vi "NavX Init.vi"(8 "error in":errorcluster) -> (0 "error out":errorcluster)   [LabVIEW 2015]
uses:
  <vilib>/Rock Robotics/SystemInterfaces/spilib/spi_bus.ctl
  Support/Global Objects.vi
  navX Library v2/IO/Open/Z900_navX_Open_SPI.vi
  navX Library v2/navX Library v2.lvlib
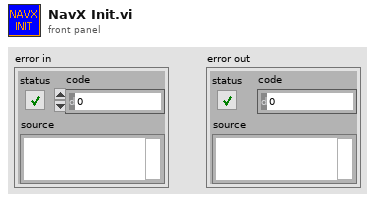
[diagram p1: front panel]
types:
  T1 = typedef "NaxX Info.ctl" = cluster{"navX Device":T2, "Current Yaw":dbl, "Active":bool}
  T2 = typedef "navX Library v2.lvlib/Z900_navX_DeviceTypeDef.ctl" = cluster{"Interface":cluster{"Protocol":T3, "Update Rate (4Hz-60Hz)":u8, "navX Open TypeDef":variant}, "Notify Packet":refnum<notifier>, "Loop VI Refnum":refnum<vi>, "Ready to Close Occurrence Refnum":refnum<k4>}
  T3 = typedef "navX Library v2.lvlib/Z900_navX_ProtocolTypeDef.ctl" = enum16{"SERIAL", "I2C", "SPI"}
  T4 = typedef "spi_bus.ctl" = enum16{"SPI On-Board, CS0", "SPI On-Board, CS1", "SPI On-Board, CS2", "SPI On-Board, CS3", "SPI MXP", "Invalid"}
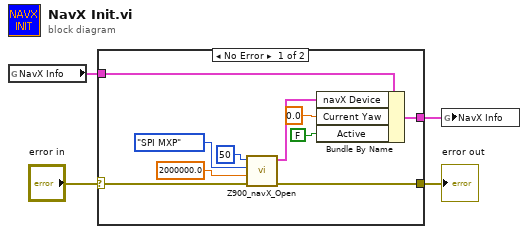
[diagram p0: block diagram]
diagram:
  n1 = global read "Global Objects.vi" "NavX Info"() -> (w2:T1)
  n2 = case shown="No Error" "error in" {
    selector: "error in" -> [w11 w16]
    tunnel: [w5 w16] -> w3
    tunnel: w2 -> [w10 w15]
    tunnel: [w9 w15] -> w1
    frame No Error {
      n3 = call-poly "Z900_navX_Open.vi"("error in (no error)"=w11, "Clock Rate (Hz)"=2000000.0, "SPI Bus"=spi_bus."SPI MXP", "Update Rate (4Hz-60Hz)"=u8 50) -> ("error out"=w5:errorcluster, "navX Device"=w6:T2)  [unwired: 6 in]
      n4 = Bundle By Name(cluster=w10, "navX Device"=w6, "Current Yaw"=0.0 ("Previous Heading"), "Active"=FALSE) -> (w9:T1)
    }
    frame Error {
    }
  }
  "error out" <- w3
  n5 = global write "Global Objects.vi" "NavX Info"(w1) -> ()
